vi "81 Arduino_Reading a voltage.vi"() -> ()   [LabVIEW 2019]
uses:
  <vilib>/Instr/_visa.llb/VISA Configure Serial Port (Instr).vi
  _Subs/OpenDiagram/Open_XControl.xctl
panel:
  in  "OpenDiag":refnum<vi>(xcontrol)
  out "Connected":bool
  in  "stop":bool
  in  "Arduino code":string="/*\n  AnalogReadSerial\n\n  Reads an analog input on pin 0, prints the result to the Serial Monitor.\n  Graphical representation is available using Serial Plotter (Tools > Serial Plotter menu).\n  Attach the center pin of a potentiometer to pin A0, and the outside pins to +5V and ground.\n\n  This example code is in the public domain.\n\n  http://www.arduino.cc/en/Tutorial/AnalogReadSerial\n*/\n\n// the setup routine runs once when you press reset:\nvoid setup() {\n  // initialize serial communication at 9600 bits per second:\n  Serial.begin(9600);\n}\n\n// the loop routine runs over and over again forever:\nvoid loop() {\n  // read the input on analog pin 0:\n  int sensorValue = analogRead(A0);\n  // print out the value you read:\n  Serial.println(sensorValue);\n  delay(1);        // delay in between reads for stability\n}"
  in  "Arduino Port":refnum<visa-resource-name>
  out "Gauge":i32(knob) scale=0.0..1000.0
  # "01 Arduino Reading a Voltage\nThis code takes will read a voltage from your Arduino\n\nInstructions:\n1. Download the Arduino Code (AnalogReadSerial) into your Arduino using the Arduino IDE\n2. Select the Arduino port \n3. Hit Run - and watch the gauge change value with the sensor"
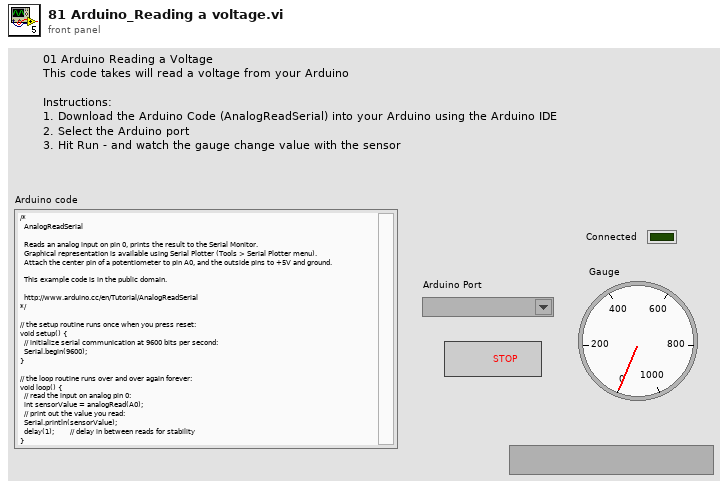
[diagram p1: front panel]
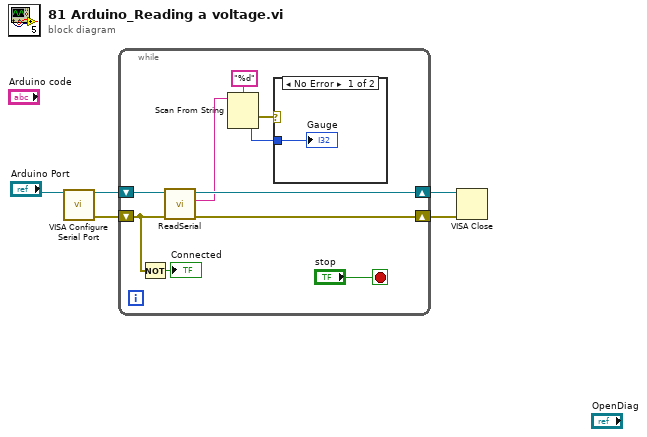
[diagram p0: block diagram]
diagram:
  n1 = call-poly "VISA Configure Serial Port"("VISA resource name"="Arduino Port") -> ("VISA resource name out"=w4:refnum<visa-resource-name>, "error out"=w3:errorcluster)  [unwired: 13 in]
  n2 = while {
    shift-right: [w13] -> w1
    shift-left: w4 -> [w15]
    shift-right: [w14] -> w2
    shift-left: w3 -> [w11]
    stop <- "stop" stop-if-true
    n3 = Not(x=w11) -> (.not. x?=→"Connected":bool)
    n4 = call "ReadSerial.vi"("error in (no error)"=w11, "VISA Refnum in"=w15) -> ("error out"=w14:errorcluster, "String"=w9:string, "VISA Refnum out"=w13:refnum<visa-resource-name>)  [unwired: 7 in]
    n5 = Scan From String(format string="%d", input string=w9) -> (error out=w8:errorcluster, output 1=w7:i32)  [unwired: 3 in, 2 out]
    n6 = case shown="No Error" w8 {
      tunnel: w7 -> [w16 _]
      frame No Error {
        "Gauge" <- w16
      }
      frame Error {
      }
    }
  }
  n7 = VISA Close(VISA resource name=w1, error in (no error)=w2) -> ()  [unwired: 1 out]
